vi "Transmit.vi"(6 "Data Input(Hex)":string="11223344556677 88", 7 "DevInd":u32, 8 "错误输入":errorcluster caption="错误输入（无错误）", 9 "ID(Hex 高位有效)":string="80000000", 10 "CANChannel":u32, 11 "DeviceType":T1=3 items=["PCI-CAN200"=7, "USB-CAN"=2, "USB-CAN200"=3]) -> (0 "错误输出":errorcluster, 1 "DeviceInd":u32, 2 "Result":bool, 3 "DeviceTypeOut":T1=3 items=["PCI-CAN200"=7, "USB-CAN"=2, "USB-CAN200"=3], 5 "CANInd":u32)   [LabVIEW 2013]
uses:
  DevType.ctl
  VCI_CAN.dll
panel:
  out "pSend":T2 {"ID" format="%02x"; "ID2" format="%02x"; "ID1" format="%02x"; "ID0" format="%02x"}
  out "VCI_CAN_OBJ_T":T3={"ID"=0, "ID2"=0, "ID1"=0, "ID0"=0, "TimeStamp"=0, "TimeFlag"=0, "SendType"=1, "RemoteFlag"=0, "ExternFlag"=0, "DataLen"=8, 0, 0, 0, 0, 0, 0, 0, 0, 0, 0, 0} {"ID0" format="%x"; "ID1" format="%x"; "ID2" format="%x"; "?" format="%02x"; "?" format="%02x"; "?" format="%02x"; "?" format="%02x"; "?" format="%02x"; "?" format="%02x"; "?" format="%02x"; "?" format="%02x"; "ID" format="%x"}
  out "Frame Format":u8(ring) items=["Data Frame", "Remote Frame"]
  out "Frame Type":u8(ring) items=["Standard Frame", "Extend Frame"]
  out "Transmit Type":u8(ring) items=["Normal Transmit"]
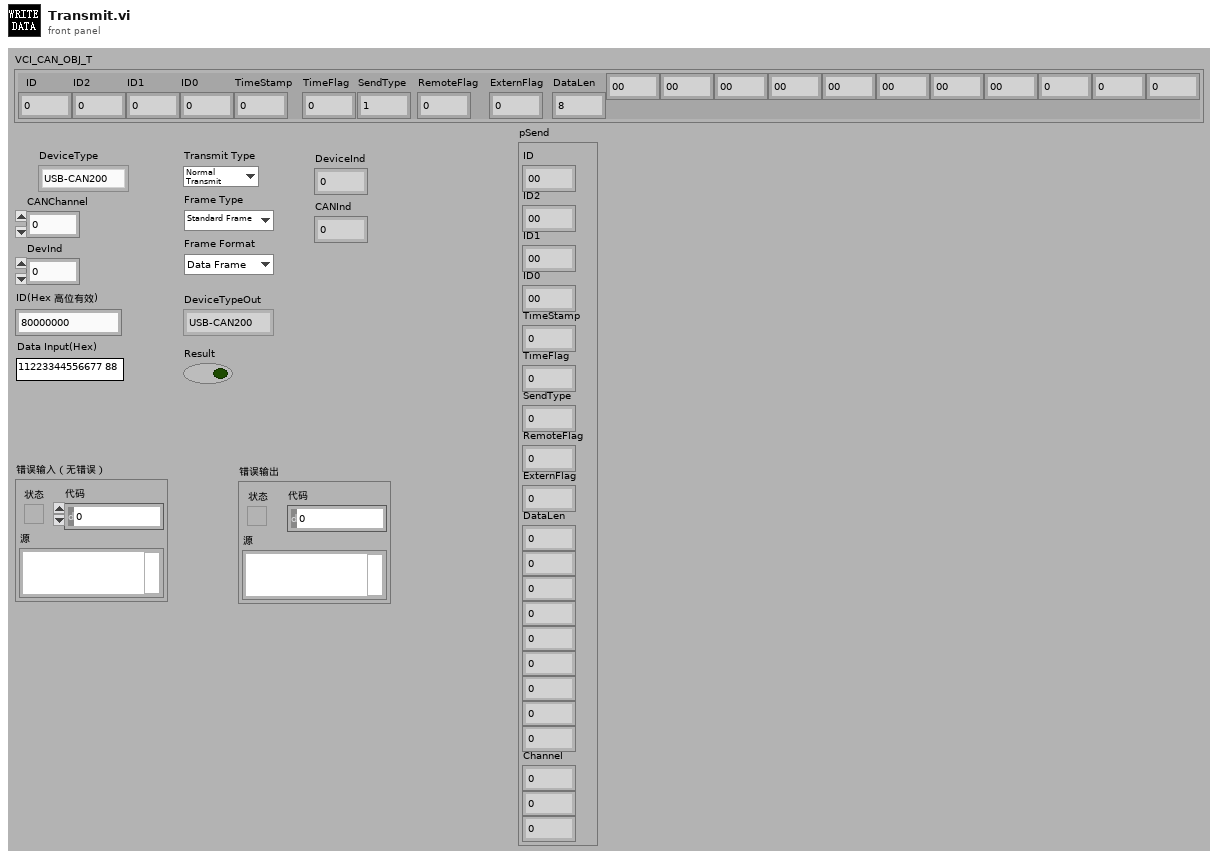
[diagram p1: front panel]
types:
  T1 = typedef "DevType.ctl" = u16
  T2 = cluster{"ID":u8, "ID2":u8, "ID1":u8, "ID0":u8, "TimeStamp":u32, "TimeFlag":u8, "SendType":u8, "RemoteFlag":u8, "ExternFlag":u8, "DataLen":u8, u8, u8, u8, u8, u8, u8, u8, u8, "Channel":u8, u8, u8}
  T3 = cluster{"ID":u8, "ID2":u8, "ID1":u8, "ID0":u8, "TimeStamp":u32, "TimeFlag":u8, "SendType":u8, "RemoteFlag":u8, "ExternFlag":u8, "DataLen":u8, u8, u8, u8, u8, u8, u8, u8, u8, u8, u8, u8}
  T4 = cluster{"Transmit Type":u8, "Frame Type":u8, "Frame Format":u8, "Data Input(Hex)":string, "ID(Hex 高位有效)":string}
  T5 = cluster{"[0]":u8, "[1]":u8, "[2]":u8, "[3]":u8, "[4]":u8, "[5]":u8, "[6]":u8, "[7]":u8, "[8]":u8}
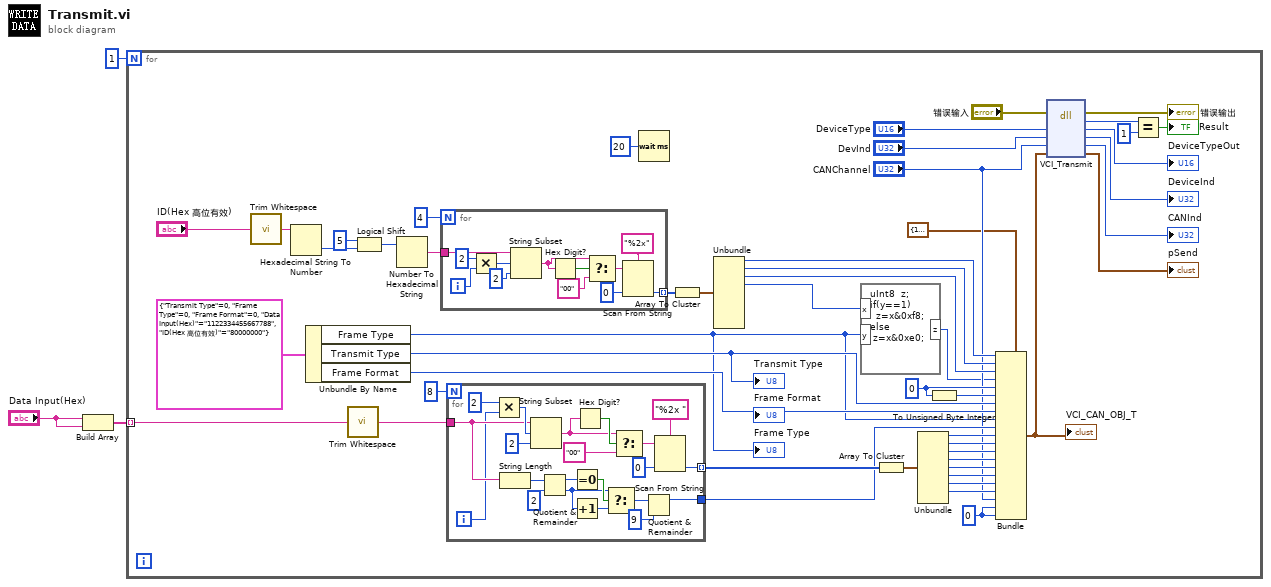
[diagram p0: block diagram]
diagram:
  n1 = Build Array("Data Input(Hex)", "Data Input(Hex)") -> (w2:string[])
  n2 = for {
    N: 1 -> [_]
    tunnel: w2 -> [w8] mode=indexing
    w46 = u8 0
    w37 = u32 0
    n3 = call <vilib>:"Trim Whitespace.vi"("string"="ID(Hex 高位有效)") -> ("trimmed string"=w10:string)  [unwired: 1 in]
    n4 = Hexadecimal String To Number(string=w10) -> (number=w13:u32)  [unwired: 2 in, 1 out]
    n5 = Unbundle By Name(T4 {"Transmit Type"=0, "Frame Type"=0, "Frame Format"=0, "Data Input(Hex)"="1122334455667788", "ID(Hex 高位有效)"="80000000"} ("CanParas")) -> ("Frame Type"=w19:u8, "Transmit Type"=w24:u8, "Frame Format"=w23:u8)
    "Transmit Type" <- w24
    "Frame Type" <- w19
    "Frame Format" <- w23
    n6 = call <vilib>:"Trim Whitespace.vi"("string"=w8) -> ("trimmed string"=w15:string)  [unwired: 1 in]
    n7 = Logical Shift(y=i8 5, x=w13) -> (x << y=w11:u32)
    n8 = Number To Hexadecimal String(2:w11) -> (0:w9:string)  [unwired: 1 in]
    n9 = for {
      N: 4 -> [_]
      tunnel: w9 -> [w56]
      tunnel: [w55] -> w30 mode=indexing
      i -> [w62]
      n10 = Multiply(x=2, y=w62) -> (x*y=w60:i32)
      n11 = String Subset(string=w56, offset (0)=w60, length (rest)=2) -> (substring=w58:string)
      n12 = Hex Digit?(1:w58) -> (0:w57:bool)
      n13 = Select(t=w58, s=w57, f="00") -> (s? t:f=w59:string)
      n14 = Scan From String(format string="%2x", input string=w59, default 1=u8 0 ("默认值 1")) -> (output 1=w55:u8)  [unwired: 2 in, 3 out]
    }
    n15 = for {
      N: 8 -> [_]
      tunnel: w15 -> [w79]
      tunnel: [w82] -> w35 mode=indexing
      tunnel: [w67] -> w33
      i -> [w72]
      n16 = Multiply(x=2, y=w72) -> (x*y=w85:i32)
      n17 = String Length(string=w79) -> (length=w78:i32)
      n18 = String Subset(string=w79, offset (0)=w85, length (rest)=2 ("length (rest)")) -> (substring=w76:string)
      n19 = Quotient & Remainder(x=w78, y=2) -> (x-y*floor(x/y)=w74:i32, floor(x/y)=w70:i32)
      n20 = Equal To 0?(x=w74) -> (x = 0?=w73:bool)
      n21 = Increment(x=w70) -> (x+1=w71:i32)
      n22 = Hex Digit?(1:w76) -> (0:w80:bool)
      n23 = Select(t=w70, s=w73, f=w71) -> (s? t:f=w69:i32)
      n24 = Select(t=w76, s=w80, f="00" ("t")) -> (s? t:f=w81:string)
      n25 = Quotient & Remainder(x=w69, y=9) -> (x-y*floor(x/y)=w67:i32)  [unwired: 1 out]
      n26 = Scan From String(format string="%2x ", input string=w81, default 1=u8 0 ("默认值 1")) -> (output 1=w82:u8)  [unwired: 2 in, 3 out]
    }
    n27 = Wait (ms)(milliseconds to wait=u32 20 ("等待时间（毫秒）")) -> ()  [unwired: 1 out]
    n28 = Array To Cluster(array=w30) -> (cluster=w29:T5)
    n29 = Unbundle(w29) -> ("[0]"=w28:u8, "[1]"=w27:u8, "[2]"=w26:u8, "[3]"=w18:u8)  [unwired: 5 out]
    n30 = formula code="uInt8  z; \nif(y==1)\n  z=x&0xf8;\nelse\n z=x&0xe0;"("x"=w18, "y"=w19) -> ("z"=w16:u8)
    n31 = Array To Cluster(array=w35) -> (cluster=w34:T5)
    n32 = Unbundle(w34) -> ("[0]"=w38:u8, "[1]"=w39:u8, "[2]"=w40:u8, "[3]"=w41:u8, "[4]"=w42:u8, "[5]"=w43:u8, "[6]"=w44:u8, "[7]"=w45:u8)  [unwired: 1 out]
    n33 = To Unsigned Byte Integer(number=w37) -> (unsigned 8bit integer=w36:u8)
    n34 = Bundle(cluster=T2 {"ID"=128, "ID2"=0, "ID1"=0, "ID0"=0, "TimeStamp"=0, "TimeFlag"=0, "SendType"=0, "RemoteFlag"=0, "ExternFlag"=0, "DataLen"=8, 17, 34, 51, 68, 85, 102, 119, 136, "Channel"=1, 0, 0} ("VCI_CAN_OBJ_T 2"), "ID"=w28, "ID2"=w27, "ID1"=w26, "ID0"=w16, "TimeStamp"=w37, "TimeFlag"=w36, "SendType"=w24, "RemoteFlag"=w23, "ExternFlag"=w19, "DataLen"=w33, w38, w39, w40, w41, w42, w43, w44, w45, "Channel"="CANChannel", w46, w46) -> (w21:T2)
    "VCI_CAN_OBJ_T" <- w21
    n35 = dll-call lib="C:/Users/Administrator/Desktop/CAN/USBCAN/VCI_CAN.dll" fn="VCI_Transmit"(error in="错误输入", "DeviceType"="DeviceType", "DeviceInd"="DevInd", "CANInd"="CANChannel", "pSend"=w21) -> (error out=→"错误输出":errorcluster, "返回类型"=w49:u32, "DeviceType"=→"DeviceTypeOut":u32, "DeviceInd"=→"DeviceInd":u32, "CANInd"=→"CANInd":u32, "pSend"=→"pSend":T2)  [unwired: 2 in, 1 out]
    n36 = Equal?(x=w49, y=u32 1) -> (x = y?=→"Result":bool)
  }
